vi "get bitfiles from files array.vi"(3 "file paths":path[](array[path])) -> (1 "FPGA bitfiles":path[](array[path]))   [LabVIEW 2014]
uses:
  <vilib>/regexp/Match Regular Expression.xnode
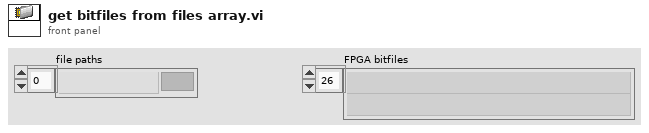
[diagram p1: front panel]
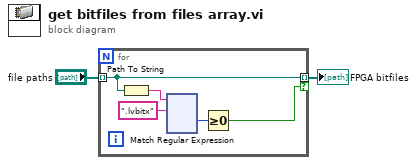
[diagram p0: block diagram]
diagram:
  n1 = for {
    tunnel: "file paths" -> [w4] mode=indexing
    tunnel: [w4] -> w1 mode=indexing if=w3
    n2 = Path To String(path=w4) -> (string=w6:string)
    n3 = xnode "Match Regular Expression"("input string"=w6, "regular expression"=".lvbitx") -> ("offset past match"=w5:i32)  [unwired: 4 in, 4 out]
    n4 = Greater Or Equal To 0?(x=w5) -> (x >= 0?=w3:bool)
  }
  "FPGA bitfiles" <- w1
